vi "メイン.vi"() -> (2 "測定周期/ms":dbl, 3 "値転記用配列":T2[](array[typedef]))   [LabVIEW 2021] (continued)
                      n747 = property on="メイン測定ボタン_単発 8" class="Bool (指定)"("BoolText.Text"=w2025) -> ()  [unwired: 2 in, 2 out]
                      n748 = local write "csv入力項目min 8"(w2019) -> ()
                      n749 = local write "csv入力項目max 8"(w2020) -> ()
                      n750 = property on="メイン測定ボタン_連続 8" class="Bool (指定)"("Visible"=w2024) -> ()  [unwired: 2 in, 2 out]
                      n751 = property on="メイン測定ボタン_単発 8" class="Bool (指定)"("Visible"=w2023) -> ()  [unwired: 2 in, 2 out]
                    }
                    frame #2 {
                      # "⑯"
                      # "⑨"
                      # "⑧"
                      # "⑦"
                      # "⑥"
                      n752 = local read "メインON/OFF_\n設定 8"() -> (w2073:T1)
                      n753 = local write "メインON/OFF_\n保存確認 8"(w2073) -> ()
                      n754 = local read "メイン設定_設定 8"() -> (w2071:T2)
                      n755 = Unbundle By Name(w2071) -> ("測定画面表示ボタン"=w2070:bool)
                      n756 = case shown="FALSE" w2070 {
                        tunnel: [w2076 TRUE] -> w2072
                        frame False {
                          w2076 = FALSE
                          n757 = property on="メイン測定ボタン_単発 8" class="Bool (指定)"("Visible"=w2076) -> ()  [unwired: 2 in, 2 out]
                          n758 = property on="メイン測定ボタン_連続 8" class="Bool (指定)"("Visible"=w2076) -> ()  [unwired: 2 in, 2 out]
                        }
                        frame True {
                        }
                      }
                      n759 = local write "メインON/OFF_制御器 8"(w2073) -> ()
                      n760 = property on="メインON/OFF_制御器 8" class="Clust (指定)"("Visible"=w2072) -> ()  [unwired: 2 in, 2 out]
                      n761 = property on="メイン設定No_設定 8" class="Clust (指定)"("Visible"=w2072) -> ()  [unwired: 2 in, 2 out]
                      n762 = property on="メイン設定_設定 8" class="Clust (指定)"("Visible"=w2072) -> ()  [unwired: 2 in, 2 out]
                      n763 = property on="キャンセルボタン 8" class="Bool (指定)"("Visible"=w2072) -> ()  [unwired: 2 in, 2 out]
                    }
                  }
                  n764 = Replace Array Subset(array=w1852, new element=w1845, index=7) -> (w1851:T2[])
                }
                frame 8 {
                  # "⑱"
                  # "⑰"
                  # "2つ目の配列に転記"
                  # "32回繰り返す為、増やす場合はこのケースストラクチャーを複製する\n複製時、設定項目の配列やボタンも複製する為、下記のボタン類の移動はしない事"
                  # "iniからデータ読み取り"
                  n765 = flat-sequence {
                    tunnel: w2087 -> [w2113]
                    tunnel: w2086 -> [w2114]
                    tunnel: [w2091] -> w2083
                    tunnel: [w2090] -> w2082
                    tunnel: w2083 -> [w2260]
                    tunnel: w2082 -> [w2259]
                    tunnel: [w2260] -> w2081
                    tunnel: [w2259] -> w2080
                    tunnel: [w2307] -> w2088
                    tunnel: [w2308] -> w2089
                    tunnel: w2081 -> [w2308]
                    tunnel: w2080 -> [w2307]
                    tunnel: [w2304] -> w2078
                    frame #0 {
                      w2092 = "設定9"
                      # "複製時に変更する項目\n①②③④⑤⑥⑦⑧⑨　⑪⑫\nローカル変数\n⑬⑭\nセレクション\n⑮⑯\nプロパティノードが\n対象配列になっているか確認\n⑰\n指標値\n⑱\n複製したケースのTrue定数を削除"
                      # "⑭"
                      # "⑬"
                      # "⑫"
                      # "⑪"
                      # "④"
                      # "③"
                      # "setting.iniファイルからの設定項目の読み取り"
                      n766 = local read "メイン設定No_設定 9"() -> (w2110:T5)
                      n767 = call-poly <vilib>:"Read Key.vi"("section"="No9.", "error in (no error)"=w2114, "key"="No.", "refnum"=w2113) -> ("error out"=w2107:errorcluster, "value"=w2111:i32, "refnum out"=w2105:T10)  [unwired: 4 in, 1 out]
                      n768 = Bundle By Name(cluster=w2110, "No."=w2111) -> (w2112:T5)
                      n769 = local write "メイン設定No_設定 9"(w2112) -> ()
                      n770 = for {
                        shift-right: [w2122] -> w2109
                        shift-left: w2105 -> [w2123]
                        shift-right: [w2119] -> w2108
                        shift-left: w2107 -> [w2120]
                        tunnel: string[] ["規格", "規格上限", "規格下限", "ポートNo.", "測定モード", "規格単位", "品質チェック項目", "測定周期", "実測MAX", "実測MIN", "実測(MAX)", "実測(MIN)", "測定画面表示ボタン", "ゲージポートNo."] -> [w2118] mode=indexing
                        tunnel: w2092 -> [w2115]
                        i -> [w2121]
                        # "②"
                        # "①"
                        n771 = local read "メイン設定_設定 9"() -> (w2116:T2)
                        n772 = case shown="0, デフォルト" w2121 {
                          tunnel: w2123 -> [w2132 w2141 w2150 w2159 w2168 w2177 w2186 w2195 w2204 w2213 w2222 w2231 w2240 w2249]
                          tunnel: [w2131 w2140 w2149 w2158 w2167 w2176 w2185 w2194 w2203 w2212 w2221 w2230 w2239 w2248] -> w2122
                          tunnel: w2115 -> [w2130 w2139 w2148 w2157 w2166 w2175 w2184 w2193 w2202 w2211 w2220 w2229 w2238 w2247]
                          tunnel: w2120 -> [w2129 w2138 w2147 w2156 w2165 w2174 w2183 w2192 w2201 w2210 w2219 w2228 w2237 w2246]
                          tunnel: [w2128 w2137 w2146 w2155 w2164 w2173 w2182 w2191 w2200 w2209 w2218 w2227 w2236 w2245] -> w2119
                          tunnel: w2118 -> [_ _ _ _ _ w2171 _ _ _ _ _ _ _ _]
                          tunnel: w2118 -> [_ _ _ _ _ _ w2180 _ _ _ _ w2225 _ _]
                          tunnel: w2118 -> [w2126 w2135 w2144 w2153 w2162 _ _ w2189 w2198 w2207 w2216 _ w2234 w2243]
                          tunnel: [w2125 w2134 w2143 w2152 w2161 w2169 w2178 w2187 w2197 w2206 w2215 w2224 w2233 w2242] -> w2117
                          tunnel: w2116 -> [w2124 w2133 w2142 w2151 w2160 w2170 w2179 w2188 w2196 w2205 w2214 w2223 w2232 w2241]
                          frame 0, Default {
                            n773 = call-poly <vilib>:"Read Key.vi"("section"=w2130, "error in (no error)"=w2129, "key"=w2126, "refnum"=w2132) -> ("error out"=w2128:errorcluster, "value"=w2127:string, "refnum out"=w2131:T10)  [unwired: 4 in, 1 out]
                            n774 = Bundle By Name(cluster=w2124, "規格"=w2127) -> (w2125:T2)
                          }
                          frame 1 {
                            n775 = call-poly <vilib>:"Read Key.vi"("section"=w2139, "error in (no error)"=w2138, "key"=w2135, "refnum"=w2141) -> ("error out"=w2137:errorcluster, "value"=w2136:string, "refnum out"=w2140:T10)  [unwired: 4 in, 1 out]
                            n776 = Bundle By Name(cluster=w2133, "規格上限"=w2136) -> (w2134:T2)
                          }
                          frame 2 {
                            n777 = call-poly <vilib>:"Read Key.vi"("section"=w2148, "error in (no error)"=w2147, "key"=w2144, "refnum"=w2150) -> ("error out"=w2146:errorcluster, "value"=w2145:string, "refnum out"=w2149:T10)  [unwired: 4 in, 1 out]
                            n778 = Bundle By Name(cluster=w2142, "規格下限"=w2145) -> (w2143:T2)
                          }
                          frame 3 {
                            n779 = call-poly <vilib>:"Read Key.vi"("section"=w2157, "error in (no error)"=w2156, "key"=w2153, "refnum"=w2159) -> ("error out"=w2155:errorcluster, "value"=w2154:i32, "refnum out"=w2158:T10)  [unwired: 4 in, 1 out]
                            n780 = Bundle By Name(cluster=w2151, "ポートNo."=w2154) -> (w2152:T2)
                          }
                          frame 4 {
                            n781 = call-poly <vilib>:"Read Key.vi"("section"=w2166, "error in (no error)"=w2165, "key"=w2162, "refnum"=w2168) -> ("error out"=w2164:errorcluster, "value"=w2163:i32, "refnum out"=w2167:T10)  [unwired: 4 in, 1 out]
                            n782 = Bundle By Name(cluster=w2160, "測定モード"=w2163) -> (w2161:T2)
                          }
                          frame 5 {
                            n783 = call-poly <vilib>:"Read Key.vi"("section"=w2175, "error in (no error)"=w2174, "key"=w2171, "refnum"=w2177) -> ("error out"=w2173:errorcluster, "value"=w2172:string, "refnum out"=w2176:T10)  [unwired: 4 in, 1 out]
                            n784 = Bundle By Name(cluster=w2170, "規格単位"=w2172) -> (w2169:T2)
                          }
                          frame 6 {
                            n785 = call-poly <vilib>:"Read Key.vi"("section"=w2184, "error in (no error)"=w2183, "key"=w2180, "refnum"=w2186) -> ("error out"=w2182:errorcluster, "value"=w2181:string, "refnum out"=w2185:T10)  [unwired: 4 in, 1 out]
                            n786 = Bundle By Name(cluster=w2179, "品質チェック項目"=w2181) -> (w2178:T2)
                          }
                          frame 7 {
                            n787 = call-poly <vilib>:"Read Key.vi"("section"=w2193, "error in (no error)"=w2192, "key"=w2189, "refnum"=w2195) -> ("error out"=w2191:errorcluster, "value"=w2190:i32, "refnum out"=w2194:T10)  [unwired: 4 in, 1 out]
                            n788 = Bundle By Name(cluster=w2188, "測定周期"=w2190) -> (w2187:T2)
                          }
                          frame 8 {
                            n789 = call-poly <vilib>:"Read Key.vi"("section"=w2202, "error in (no error)"=w2201, "key"=w2198, "refnum"=w2204) -> ("error out"=w2200:errorcluster, "value"=w2199:string, "refnum out"=w2203:T10)  [unwired: 4 in, 1 out]
                            n790 = Bundle By Name(cluster=w2196, "実測値MAX"=w2199) -> (w2197:T2)
                          }
                          frame 9 {
                            n791 = call-poly <vilib>:"Read Key.vi"("section"=w2211, "error in (no error)"=w2210, "key"=w2207, "refnum"=w2213) -> ("error out"=w2209:errorcluster, "value"=w2208:string, "refnum out"=w2212:T10)  [unwired: 4 in, 1 out]
                            n792 = Bundle By Name(cluster=w2205, "実測値MIN"=w2208) -> (w2206:T2)
                          }
                          frame 10 {
                            n793 = call-poly <vilib>:"Read Key.vi"("section"=w2220, "error in (no error)"=w2219, "key"=w2216, "refnum"=w2222) -> ("error out"=w2218:errorcluster, "value"=w2217:string, "refnum out"=w2221:T10)  [unwired: 4 in, 1 out]
                            n794 = Bundle By Name(cluster=w2214, "実測値(MAX)"=w2217) -> (w2215:T2)
                          }
                          frame 11 {
                            n795 = call-poly <vilib>:"Read Key.vi"("section"=w2229, "error in (no error)"=w2228, "key"=w2225, "refnum"=w2231) -> ("error out"=w2227:errorcluster, "value"=w2226:string, "refnum out"=w2230:T10)  [unwired: 4 in, 1 out]
                            n796 = Bundle By Name(cluster=w2223, "実測値(MIN)"=w2226) -> (w2224:T2)
                          }
                          frame 12 {
                            n797 = call-poly <vilib>:"Read Key.vi"("section"=w2238, "error in (no error)"=w2237, "key"=w2234, "refnum"=w2240) -> ("error out"=w2236:errorcluster, "value"=w2235:bool, "refnum out"=w2239:T10)  [unwired: 4 in, 1 out]
                            n798 = Bundle By Name(cluster=w2232, "測定画面表示ボタン"=w2235) -> (w2233:T2)
                          }
                          frame 13 {
                            n799 = call-poly <vilib>:"Read Key.vi"("section"=w2247, "error in (no error)"=w2246, "key"=w2243, "refnum"=w2249) -> ("error out"=w2245:errorcluster, "value"=w2244:string, "refnum out"=w2248:T10)  [unwired: 4 in, 1 out]
                            n800 = Bundle By Name(cluster=w2241, "ゲージポートNo"=w2244) -> (w2242:T2)
                          }
                        }
                        n801 = local write "メイン設定_設定 9"(w2117) -> ()
                      }
                      n802 = local read "メインON/OFF_\n設定 9"() -> (w2101:T1)
                      n803 = call-poly <vilib>:"Read Key.vi"("section"=w2092, "error in (no error)"=w2108, "key"="使用ON/OFF", "refnum"=w2109) -> ("error out"=w2093:errorcluster, "value"=w2099:bool, "refnum out"=w2094:T10)  [unwired: 4 in, 1 out]
                      n804 = Bundle By Name(cluster=w2101, "使用ON/OFF"=w2099) -> (w2102:T1)
                      n805 = local write "メインON/OFF_\n設定 9"(w2102) -> ()
                      n806 = local read "CSV項目名 9"() -> (w2097:T3)
                      n807 = call-poly <vilib>:"Read Key.vi"("section"=w2092, "error in (no error)"=w2093, "key"="CSVヘッダー名", "refnum"=w2094) -> ("error out"=w2090:errorcluster, "value"=w2095:string, "refnum out"=w2091:T10)  [unwired: 4 in, 1 out]
                      n808 = Bundle By Name(cluster=w2097, "CSV項目名"=w2095) -> (w2096:T3)
                      n809 = local write "CSV項目名 9"(w2096) -> ()
                    }
                    frame #1 {
                      # "csvヘッダー項目作成"
                      # "⑮"
                      # "⑤"
                      n810 = local read "CSV項目名 9"() -> (w2254:T3)
                      n811 = Unbundle By Name(w2254) -> ("CSV項目名"=w2251:string)
                      n812 = local read "メイン設定_設定 9"() -> (w2255:T2)
                      n813 = Unbundle By Name(w2255) -> ("測定モード"=w2250:u16)
                      n814 = case shown="0, デフォルト" w2250 {
                        tunnel: ["単発測定" _ "多点測定"] -> w2258
                        tunnel: [FALSE TRUE FALSE] -> w2257
                        tunnel: [TRUE FALSE TRUE] -> w2256
                        frame 0, Default {
                        }
                        frame 1 {
                        }
                        frame 2 {
                        }
                      }
                      n815 = case shown="1" w2250 {
                        tunnel: w2251 -> [w2264 w2276 w2285]
                        tunnel: [w2262 w2274 w2287] -> w2253
                        tunnel: [w2261 w2273 w2286] -> w2252
                        frame 1 {
                          n816 = Empty String/Path?(string/path=w2264) -> (empty?=w2263:bool)
                          n817 = case shown="FALSE" w2263 {
                            tunnel: w2264 -> [w2270 _]
                            tunnel: w2264 -> [w2269 _]
                            tunnel: [w2266 ""] -> w2262
                            tunnel: [w2265 ""] -> w2261
                            frame False {
                              n818 = Concatenate Strings(w2270, "_max") -> (w2266:string)
                              n819 = Concatenate Strings(w2269, "_min") -> (w2265:string)
                            }
                            frame True {
                            }
                          }
                        }
                        frame 2 {
                          n820 = Empty String/Path?(string/path=w2276) -> (empty?=w2275:bool)
                          n821 = case shown="FALSE" w2275 {
                            tunnel: w2276 -> [w2282 _]
                            tunnel: w2276 -> [w2281 _]
                            tunnel: [w2278 ""] -> w2274
                            tunnel: [w2277 ""] -> w2273
                            frame False {
                              n822 = Concatenate Strings(w2282, "_max") -> (w2278:string)
                              n823 = Concatenate Strings(w2281, "_min") -> (w2277:string)
                            }
                            frame True {
                            }
                          }
                        }
                        frame 0, Default {
                          n824 = Empty String/Path?(string/path=w2285) -> (empty?=w2288:bool)
                          n825 = case shown="FALSE" w2288 {
                            tunnel: w2285 -> [w2292 _]
                            tunnel: [w2290 ""] -> w2287
                            tunnel: ["" ""] -> w2286
                            frame False {
                              n826 = Concatenate Strings(w2292, "_value") -> (w2290:string)
                            }
                            frame True {
                            }
                          }
                        }
                      }
                      n827 = property on="メイン測定ボタン_単発 9" class="Bool (指定)"("BoolText.Text"=w2258) -> ()  [unwired: 2 in, 2 out]
                      n828 = local write "csv入力項目min 9"(w2252) -> ()
                      n829 = local write "csv入力項目max 9"(w2253) -> ()
                      n830 = property on="メイン測定ボタン_連続 9" class="Bool (指定)"("Visible"=w2257) -> ()  [unwired: 2 in, 2 out]
                      n831 = property on="メイン測定ボタン_単発 9" class="Bool (指定)"("Visible"=w2256) -> ()  [unwired: 2 in, 2 out]
                    }
                    frame #2 {
                      # "⑯"
                      # "⑨"
                      # "⑧"
                      # "⑦"
                      # "⑥"
                      n832 = local read "メインON/OFF_\n設定 9"() -> (w2306:T1)
                      n833 = local write "メインON/OFF_\n保存確認 9"(w2306) -> ()
                      n834 = local read "メイン設定_設定 9"() -> (w2304:T2)
                      n835 = Unbundle By Name(w2304) -> ("測定画面表示ボタン"=w2303:bool)
                      n836 = case shown="FALSE" w2303 {
                        tunnel: [w2309 TRUE] -> w2305
                        frame False {
                          w2309 = FALSE
                          n837 = property on="メイン測定ボタン_単発 9" class="Bool (指定)"("Visible"=w2309) -> ()  [unwired: 2 in, 2 out]
                          n838 = property on="メイン測定ボタン_連続 9" class="Bool (指定)"("Visible"=w2309) -> ()  [unwired: 2 in, 2 out]
                        }
                        frame True {
                        }
                      }
                      n839 = local write "メインON/OFF_制御器 9"(w2306) -> ()
                      n840 = property on="メインON/OFF_制御器 9" class="Clust (指定)"("Visible"=w2305) -> ()  [unwired: 2 in, 2 out]
                      n841 = property on="メイン設定No_設定 9" class="Clust (指定)"("Visible"=w2305) -> ()  [unwired: 2 in, 2 out]
                      n842 = property on="メイン設定_設定 9" class="Clust (指定)"("Visible"=w2305) -> ()  [unwired: 2 in, 2 out]
                      n843 = property on="キャンセルボタン 9" class="Bool (指定)"("Visible"=w2305) -> ()  [unwired: 2 in, 2 out]
                    }
                  }
                  n844 = Replace Array Subset(array=w2085, new element=w2078, index=8) -> (w2084:T2[])
                }
                frame 9 {
                  # "⑱"
                  # "⑰"
                  # "2つ目の配列に転記"
                  # "32回繰り返す為、増やす場合はこのケースストラクチャーを複製する\n複製時、設定項目の配列やボタンも複製する為、下記のボタン類の移動はしない事"
                  # "iniからデータ読み取り"
                  n845 = flat-sequence {
                    tunnel: w2320 -> [w2346]
                    tunnel: w2319 -> [w2347]
                    tunnel: [w2325] -> w2316
                    tunnel: [w2324] -> w2315
                    tunnel: w2316 -> [w2493]
                    tunnel: w2315 -> [w2492]
                    tunnel: [w2493] -> w2314
                    tunnel: [w2492] -> w2313
                    tunnel: [w2540] -> w2321
                    tunnel: [w2541] -> w2322
                    tunnel: w2314 -> [w2541]
                    tunnel: w2313 -> [w2540]
                    tunnel: [w2537] -> w2311
                    frame #0 {
                      w2323 = "設定10"
                      # "複製時に変更する項目\n①②③④⑤⑥⑦⑧⑨　⑪⑫\nローカル変数\n⑬⑭\nセレクション\n⑮⑯\nプロパティノードが\n対象配列になっているか確認\n⑰\n指標値\n⑱\n複製したケースのTrue定数を削除"
                      # "⑭"
                      # "⑬"
                      # "⑫"
                      # "⑪"
                      # "④"
                      # "③"
                      # "setting.iniファイルからの設定項目の読み取り"
                      n846 = local read "メイン設定No_設定 10"() -> (w2343:T5)
                      n847 = call-poly <vilib>:"Read Key.vi"("section"="No10.", "error in (no error)"=w2347, "key"="No.", "refnum"=w2346) -> ("error out"=w2340:errorcluster, "value"=w2344:i32, "refnum out"=w2338:T10)  [unwired: 4 in, 1 out]
                      n848 = Bundle By Name(cluster=w2343, "No."=w2344) -> (w2345:T5)
                      n849 = local write "メイン設定No_設定 10"(w2345) -> ()
                      n850 = for {
                        shift-right: [w2355] -> w2342
                        shift-left: w2338 -> [w2356]
                        shift-right: [w2352] -> w2341
                        shift-left: w2340 -> [w2353]
                        tunnel: string[] ["規格", "規格上限", "規格下限", "ポートNo.", "測定モード", "規格単位", "品質チェック項目", "測定周期", "実測MAX", "実測MIN", "実測(MAX)", "実測(MIN)", "測定画面表示ボタン", "ゲージポートNo."] -> [w2351] mode=indexing
                        tunnel: w2323 -> [w2348]
                        i -> [w2354]
                        # "②"
                        # "①"
                        n851 = local read "メイン設定_設定 10"() -> (w2349:T2)
                        n852 = case shown="0, デフォルト" w2354 {
                          tunnel: w2356 -> [w2365 w2374 w2383 w2392 w2401 w2410 w2419 w2428 w2437 w2446 w2455 w2464 w2473 w2482]
                          tunnel: [w2364 w2373 w2382 w2391 w2400 w2409 w2418 w2427 w2436 w2445 w2454 w2463 w2472 w2481] -> w2355
                          tunnel: w2348 -> [w2363 w2372 w2381 w2390 w2399 w2408 w2417 w2426 w2435 w2444 w2453 w2462 w2471 w2480]
                          tunnel: w2353 -> [w2362 w2371 w2380 w2389 w2398 w2407 w2416 w2425 w2434 w2443 w2452 w2461 w2470 w2479]
                          tunnel: [w2361 w2370 w2379 w2388 w2397 w2406 w2415 w2424 w2433 w2442 w2451 w2460 w2469 w2478] -> w2352
                          tunnel: w2351 -> [_ _ _ _ _ w2404 _ _ _ _ _ _ _ _]
                          tunnel: w2351 -> [_ _ _ _ _ _ w2413 _ _ _ _ w2458 _ _]
                          tunnel: w2351 -> [w2359 w2368 w2377 w2386 w2395 _ _ w2422 w2431 w2440 w2449 _ w2467 w2476]
                          tunnel: [w2358 w2367 w2376 w2385 w2394 w2402 w2411 w2420 w2430 w2439 w2448 w2457 w2466 w2475] -> w2350
                          tunnel: w2349 -> [w2357 w2366 w2375 w2384 w2393 w2403 w2412 w2421 w2429 w2438 w2447 w2456 w2465 w2474]
                          frame 0, Default {
                            n853 = call-poly <vilib>:"Read Key.vi"("section"=w2363, "error in (no error)"=w2362, "key"=w2359, "refnum"=w2365) -> ("error out"=w2361:errorcluster, "value"=w2360:string, "refnum out"=w2364:T10)  [unwired: 4 in, 1 out]
                            n854 = Bundle By Name(cluster=w2357, "規格"=w2360) -> (w2358:T2)
                          }
                          frame 1 {
                            n855 = call-poly <vilib>:"Read Key.vi"("section"=w2372, "error in (no error)"=w2371, "key"=w2368, "refnum"=w2374) -> ("error out"=w2370:errorcluster, "value"=w2369:string, "refnum out"=w2373:T10)  [unwired: 4 in, 1 out]
                            n856 = Bundle By Name(cluster=w2366, "規格上限"=w2369) -> (w2367:T2)
                          }
                          frame 2 {
                            n857 = call-poly <vilib>:"Read Key.vi"("section"=w2381, "error in (no error)"=w2380, "key"=w2377, "refnum"=w2383) -> ("error out"=w2379:errorcluster, "value"=w2378:string, "refnum out"=w2382:T10)  [unwired: 4 in, 1 out]
                            n858 = Bundle By Name(cluster=w2375, "規格下限"=w2378) -> (w2376:T2)
                          }
                          frame 3 {
                            n859 = call-poly <vilib>:"Read Key.vi"("section"=w2390, "error in (no error)"=w2389, "key"=w2386, "refnum"=w2392) -> ("error out"=w2388:errorcluster, "value"=w2387:i32, "refnum out"=w2391:T10)  [unwired: 4 in, 1 out]
                            n860 = Bundle By Name(cluster=w2384, "ポートNo."=w2387) -> (w2385:T2)
                          }
                          frame 4 {
                            n861 = call-poly <vilib>:"Read Key.vi"("section"=w2399, "error in (no error)"=w2398, "key"=w2395, "refnum"=w2401) -> ("error out"=w2397:errorcluster, "value"=w2396:i32, "refnum out"=w2400:T10)  [unwired: 4 in, 1 out]
                            n862 = Bundle By Name(cluster=w2393, "測定モード"=w2396) -> (w2394:T2)
                          }
                          frame 5 {
                            n863 = call-poly <vilib>:"Read Key.vi"("section"=w2408, "error in (no error)"=w2407, "key"=w2404, "refnum"=w2410) -> ("error out"=w2406:errorcluster, "value"=w2405:string, "refnum out"=w2409:T10)  [unwired: 4 in, 1 out]
                            n864 = Bundle By Name(cluster=w2403, "規格単位"=w2405) -> (w2402:T2)
                          }
                          frame 6 {
                            n865 = call-poly <vilib>:"Read Key.vi"("section"=w2417, "error in (no error)"=w2416, "key"=w2413, "refnum"=w2419) -> ("error out"=w2415:errorcluster, "value"=w2414:string, "refnum out"=w2418:T10)  [unwired: 4 in, 1 out]
                            n866 = Bundle By Name(cluster=w2412, "品質チェック項目"=w2414) -> (w2411:T2)
                          }
                          frame 7 {
                            n867 = call-poly <vilib>:"Read Key.vi"("section"=w2426, "error in (no error)"=w2425, "key"=w2422, "refnum"=w2428) -> ("error out"=w2424:errorcluster, "value"=w2423:i32, "refnum out"=w2427:T10)  [unwired: 4 in, 1 out]
                            n868 = Bundle By Name(cluster=w2421, "測定周期"=w2423) -> (w2420:T2)
                          }
                          frame 8 {
                            n869 = call-poly <vilib>:"Read Key.vi"("section"=w2435, "error in (no error)"=w2434, "key"=w2431, "refnum"=w2437) -> ("error out"=w2433:errorcluster, "value"=w2432:string, "refnum out"=w2436:T10)  [unwired: 4 in, 1 out]
                            n870 = Bundle By Name(cluster=w2429, "実測値MAX"=w2432) -> (w2430:T2)
                          }
                          frame 9 {
                            n871 = call-poly <vilib>:"Read Key.vi"("section"=w2444, "error in (no error)"=w2443, "key"=w2440, "refnum"=w2446) -> ("error out"=w2442:errorcluster, "value"=w2441:string, "refnum out"=w2445:T10)  [unwired: 4 in, 1 out]
                            n872 = Bundle By Name(cluster=w2438, "実測値MIN"=w2441) -> (w2439:T2)
                          }
                          frame 10 {
                            n873 = call-poly <vilib>:"Read Key.vi"("section"=w2453, "error in (no error)"=w2452, "key"=w2449, "refnum"=w2455) -> ("error out"=w2451:errorcluster, "value"=w2450:string, "refnum out"=w2454:T10)  [unwired: 4 in, 1 out]
                            n874 = Bundle By Name(cluster=w2447, "実測値(MAX)"=w2450) -> (w2448:T2)
                          }
                          frame 11 {
                            n875 = call-poly <vilib>:"Read Key.vi"("section"=w2462, "error in (no error)"=w2461, "key"=w2458, "refnum"=w2464) -> ("error out"=w2460:errorcluster, "value"=w2459:string, "refnum out"=w2463:T10)  [unwired: 4 in, 1 out]
                            n876 = Bundle By Name(cluster=w2456, "実測値(MIN)"=w2459) -> (w2457:T2)
                          }
                          frame 12 {
                            n877 = call-poly <vilib>:"Read Key.vi"("section"=w2471, "error in (no error)"=w2470, "key"=w2467, "refnum"=w2473) -> ("error out"=w2469:errorcluster, "value"=w2468:bool, "refnum out"=w2472:T10)  [unwired: 4 in, 1 out]
                            n878 = Bundle By Name(cluster=w2465, "測定画面表示ボタン"=w2468) -> (w2466:T2)
                          }
                          frame 13 {
                            n879 = call-poly <vilib>:"Read Key.vi"("section"=w2480, "error in (no error)"=w2479, "key"=w2476, "refnum"=w2482) -> ("error out"=w2478:errorcluster, "value"=w2477:string, "refnum out"=w2481:T10)  [unwired: 4 in, 1 out]
                            n880 = Bundle By Name(cluster=w2474, "ゲージポートNo"=w2477) -> (w2475:T2)
                          }
                        }
                        n881 = local write "メイン設定_設定 10"(w2350) -> ()
                      }
                      n882 = local read "メインON/OFF_\n設定 10"() -> (w2334:T1)
                      n883 = call-poly <vilib>:"Read Key.vi"("section"=w2323, "error in (no error)"=w2341, "key"="使用ON/OFF", "refnum"=w2342) -> ("error out"=w2326:errorcluster, "value"=w2332:bool, "refnum out"=w2327:T10)  [unwired: 4 in, 1 out]
                      n884 = Bundle By Name(cluster=w2334, "使用ON/OFF"=w2332) -> (w2335:T1)
                      n885 = local write "メインON/OFF_\n設定 10"(w2335) -> ()
                      n886 = local read "CSV項目名 10"() -> (w2330:T3)
                      n887 = call-poly <vilib>:"Read Key.vi"("section"=w2323, "error in (no error)"=w2326, "key"="CSVヘッダー名", "refnum"=w2327) -> ("error out"=w2324:errorcluster, "value"=w2328:string, "refnum out"=w2325:T10)  [unwired: 4 in, 1 out]
                      n888 = Bundle By Name(cluster=w2330, "CSV項目名"=w2328) -> (w2329:T3)
                      n889 = local write "CSV項目名 10"(w2329) -> ()
                    }
                    frame #1 {
                      # "csvヘッダー項目作成"
                      # "⑮"
                      # "⑤"
                      n890 = local read "CSV項目名 10"() -> (w2487:T3)
                      n891 = Unbundle By Name(w2487) -> ("CSV項目名"=w2484:string)
                      n892 = local read "メイン設定_設定 10"() -> (w2488:T2)
                      n893 = Unbundle By Name(w2488) -> ("測定モード"=w2483:u16)
                      n894 = case shown="0, デフォルト" w2483 {
                        tunnel: ["単発測定" _ "多点測定"] -> w2491
                        tunnel: [FALSE TRUE FALSE] -> w2490
                        tunnel: [TRUE FALSE TRUE] -> w2489
                        frame 0, Default {
                        }
                        frame 1 {
                        }
                        frame 2 {
                        }
                      }
                      n895 = case shown="1" w2483 {
                        tunnel: w2484 -> [w2497 w2509 w2518]
                        tunnel: [w2495 w2507 w2520] -> w2486
                        tunnel: [w2494 w2506 w2519] -> w2485
                        frame 1 {
                          n896 = Empty String/Path?(string/path=w2497) -> (empty?=w2496:bool)
                          n897 = case shown="FALSE" w2496 {
                            tunnel: w2497 -> [w2503 _]
                            tunnel: w2497 -> [w2502 _]
                            tunnel: [w2499 ""] -> w2495
                            tunnel: [w2498 ""] -> w2494
                            frame False {
                              n898 = Concatenate Strings(w2503, "_max") -> (w2499:string)
                              n899 = Concatenate Strings(w2502, "_min") -> (w2498:string)
                            }
                            frame True {
                            }
                          }
                        }
                        frame 2 {
                          n900 = Empty String/Path?(string/path=w2509) -> (empty?=w2508:bool)
                          n901 = case shown="FALSE" w2508 {
                            tunnel: w2509 -> [w2515 _]
                            tunnel: w2509 -> [w2514 _]
                            tunnel: [w2511 ""] -> w2507
                            tunnel: [w2510 ""] -> w2506
                            frame False {
                              n902 = Concatenate Strings(w2515, "_max") -> (w2511:string)
                              n903 = Concatenate Strings(w2514, "_min") -> (w2510:string)
                            }
                            frame True {
                            }
                          }
                        }
                        frame 0, Default {
                          n904 = Empty String/Path?(string/path=w2518) -> (empty?=w2521:bool)
                          n905 = case shown="FALSE" w2521 {
                            tunnel: w2518 -> [w2525 _]
                            tunnel: [w2523 ""] -> w2520
                            tunnel: ["" ""] -> w2519
                            frame False {
                              n906 = Concatenate Strings(w2525, "_value") -> (w2523:string)
                            }
                            frame True {
                            }
                          }
                        }
                      }
                      n907 = property on="メイン測定ボタン_単発 10" class="Bool (指定)"("BoolText.Text"=w2491) -> ()  [unwired: 2 in, 2 out]
                      n908 = local write "csv入力項目min 10"(w2485) -> ()
                      n909 = local write "csv入力項目max 10"(w2486) -> ()
                      n910 = property on="メイン測定ボタン_連続 10" class="Bool (指定)"("Visible"=w2490) -> ()  [unwired: 2 in, 2 out]
                      n911 = property on="メイン測定ボタン_単発 10" class="Bool (指定)"("Visible"=w2489) -> ()  [unwired: 2 in, 2 out]
                    }
                    frame #2 {
                      # "⑯"
                      # "⑨"
                      # "⑧"
                      # "⑦"
                      # "⑥"
                      n912 = local read "メインON/OFF_\n設定 10"() -> (w2539:T1)
                      n913 = local write "メインON/OFF_\n保存確認 10"(w2539) -> ()
                      n914 = local read "メイン設定_設定 10"() -> (w2537:T2)
                      n915 = Unbundle By Name(w2537) -> ("測定画面表示ボタン"=w2536:bool)
                      n916 = case shown="FALSE" w2536 {
                        tunnel: [w2542 TRUE] -> w2538
                        frame False {
                          w2542 = FALSE
                          n917 = property on="メイン測定ボタン_単発 10" class="Bool (指定)"("Visible"=w2542) -> ()  [unwired: 2 in, 2 out]
                          n918 = property on="メイン測定ボタン_連続 10" class="Bool (指定)"("Visible"=w2542) -> ()  [unwired: 2 in, 2 out]
                        }
                        frame True {
                        }
                      }
                      n919 = local write "メインON/OFF_制御器 10"(w2539) -> ()
                      n920 = property on="メインON/OFF_制御器 10" class="Clust (指定)"("Visible"=w2538) -> ()  [unwired: 2 in, 2 out]
                      n921 = property on="メイン設定No_設定 10" class="Clust (指定)"("Visible"=w2538) -> ()  [unwired: 2 in, 2 out]
                      n922 = property on="メイン設定_設定 10" class="Clust (指定)"("Visible"=w2538) -> ()  [unwired: 2 in, 2 out]
                      n923 = property on="キャンセルボタン 10" class="Bool (指定)"("Visible"=w2538) -> ()  [unwired: 2 in, 2 out]
                    }
                  }
                  n924 = Replace Array Subset(array=w2318, new element=w2311, index=9) -> (w2317:T2[])
                }
                frame 10 {
                  # "⑱"
                  # "⑰"
                  # "2つ目の配列に転記"
                  # "32回繰り返す為、増やす場合はこのケースストラクチャーを複製する\n複製時、設定項目の配列やボタンも複製する為、下記のボタン類の移動はしない事"
                  # "iniからデータ読み取り"
                  n925 = flat-sequence {
                    tunnel: w2553 -> [w2579]
                    tunnel: w2552 -> [w2580]
                    tunnel: [w2557] -> w2549
                    tunnel: [w2556] -> w2548
                    tunnel: w2549 -> [w2726]
                    tunnel: w2548 -> [w2725]
                    tunnel: [w2726] -> w2547
                    tunnel: [w2725] -> w2546
                    tunnel: [w2773] -> w2554
                    tunnel: [w2774] -> w2555
                    tunnel: w2547 -> [w2774]
                    tunnel: w2546 -> [w2773]
                    tunnel: [w2770] -> w2544
                    frame #0 {
                      w2558 = "設定11"
                      # "複製時に変更する項目\n①②③④⑤⑥⑦⑧⑨　⑪⑫\nローカル変数\n⑬⑭\nセレクション\n⑮⑯\nプロパティノードが\n対象配列になっているか確認\n⑰\n指標値\n⑱\n複製したケースのTrue定数を削除"
                      # "⑭"
                      # "⑬"
                      # "⑫"
                      # "⑪"
                      # "④"
                      # "③"
                      # "setting.iniファイルからの設定項目の読み取り"
                      n926 = local read "メイン設定No_設定 11"() -> (w2576:T5)
                      n927 = call-poly <vilib>:"Read Key.vi"("section"="No11.", "error in (no error)"=w2580, "key"="No.", "refnum"=w2579) -> ("error out"=w2573:errorcluster, "value"=w2577:i32, "refnum out"=w2571:T10)  [unwired: 4 in, 1 out]
                      n928 = Bundle By Name(cluster=w2576, "No."=w2577) -> (w2578:T5)
                      n929 = local write "メイン設定No_設定 11"(w2578) -> ()
                      n930 = for {
                        shift-right: [w2588] -> w2575
                        shift-left: w2571 -> [w2589]
                        shift-right: [w2585] -> w2574
                        shift-left: w2573 -> [w2586]
                        tunnel: string[] ["規格", "規格上限", "規格下限", "ポートNo.", "測定モード", "規格単位", "品質チェック項目", "測定周期", "実測MAX", "実測MIN", "実測(MAX)", "実測(MIN)", "測定画面表示ボタン", "ゲージポートNo."] -> [w2584] mode=indexing
                        tunnel: w2558 -> [w2581]
                        i -> [w2587]
                        # "②"
                        # "①"
                        n931 = local read "メイン設定_設定 11"() -> (w2582:T2)
                        n932 = case shown="0, デフォルト" w2587 {
                          tunnel: w2589 -> [w2598 w2607 w2616 w2625 w2634 w2643 w2652 w2661 w2670 w2679 w2688 w2697 w2706 w2715]
                          tunnel: [w2597 w2606 w2615 w2624 w2633 w2642 w2651 w2660 w2669 w2678 w2687 w2696 w2705 w2714] -> w2588
                          tunnel: w2581 -> [w2596 w2605 w2614 w2623 w2632 w2641 w2650 w2659 w2668 w2677 w2686 w2695 w2704 w2713]
                          tunnel: w2586 -> [w2595 w2604 w2613 w2622 w2631 w2640 w2649 w2658 w2667 w2676 w2685 w2694 w2703 w2712]
                          tunnel: [w2594 w2603 w2612 w2621 w2630 w2639 w2648 w2657 w2666 w2675 w2684 w2693 w2702 w2711] -> w2585
                          tunnel: w2584 -> [_ _ _ _ _ w2637 _ _ _ _ _ _ _ _]
                          tunnel: w2584 -> [_ _ _ _ _ _ w2646 _ _ _ _ w2691 _ _]
                          tunnel: w2584 -> [w2592 w2601 w2610 w2619 w2628 _ _ w2655 w2664 w2673 w2682 _ w2700 w2709]
                          tunnel: [w2591 w2600 w2609 w2618 w2627 w2635 w2644 w2653 w2663 w2672 w2681 w2690 w2699 w2708] -> w2583
                          tunnel: w2582 -> [w2590 w2599 w2608 w2617 w2626 w2636 w2645 w2654 w2662 w2671 w2680 w2689 w2698 w2707]
                          frame 0, Default {
                            n933 = call-poly <vilib>:"Read Key.vi"("section"=w2596, "error in (no error)"=w2595, "key"=w2592, "refnum"=w2598) -> ("error out"=w2594:errorcluster, "value"=w2593:string, "refnum out"=w2597:T10)  [unwired: 4 in, 1 out]
                            n934 = Bundle By Name(cluster=w2590, "規格"=w2593) -> (w2591:T2)
                          }
                          frame 1 {
                            n935 = call-poly <vilib>:"Read Key.vi"("section"=w2605, "error in (no error)"=w2604, "key"=w2601, "refnum"=w2607) -> ("error out"=w2603:errorcluster, "value"=w2602:string, "refnum out"=w2606:T10)  [unwired: 4 in, 1 out]
                            n936 = Bundle By Name(cluster=w2599, "規格上限"=w2602) -> (w2600:T2)
                          }
                          frame 2 {
                            n937 = call-poly <vilib>:"Read Key.vi"("section"=w2614, "error in (no error)"=w2613, "key"=w2610, "refnum"=w2616) -> ("error out"=w2612:errorcluster, "value"=w2611:string, "refnum out"=w2615:T10)  [unwired: 4 in, 1 out]
                            n938 = Bundle By Name(cluster=w2608, "規格下限"=w2611) -> (w2609:T2)
                          }
                          frame 3 {
                            n939 = call-poly <vilib>:"Read Key.vi"("section"=w2623, "error in (no error)"=w2622, "key"=w2619, "refnum"=w2625) -> ("error out"=w2621:errorcluster, "value"=w2620:i32, "refnum out"=w2624:T10)  [unwired: 4 in, 1 out]
                            n940 = Bundle By Name(cluster=w2617, "ポートNo."=w2620) -> (w2618:T2)
                          }
                          frame 4 {
                            n941 = call-poly <vilib>:"Read Key.vi"("section"=w2632, "error in (no error)"=w2631, "key"=w2628, "refnum"=w2634) -> ("error out"=w2630:errorcluster, "value"=w2629:i32, "refnum out"=w2633:T10)  [unwired: 4 in, 1 out]
                            n942 = Bundle By Name(cluster=w2626, "測定モード"=w2629) -> (w2627:T2)
                          }
                          frame 5 {
                            n943 = call-poly <vilib>:"Read Key.vi"("section"=w2641, "error in (no error)"=w2640, "key"=w2637, "refnum"=w2643) -> ("error out"=w2639:errorcluster, "value"=w2638:string, "refnum out"=w2642:T10)  [unwired: 4 in, 1 out]
                            n944 = Bundle By Name(cluster=w2636, "規格単位"=w2638) -> (w2635:T2)
                          }
                          frame 6 {
                            n945 = call-poly <vilib>:"Read Key.vi"("section"=w2650, "error in (no error)"=w2649, "key"=w2646, "refnum"=w2652) -> ("error out"=w2648:errorcluster, "value"=w2647:string, "refnum out"=w2651:T10)  [unwired: 4 in, 1 out]
                            n946 = Bundle By Name(cluster=w2645, "品質チェック項目"=w2647) -> (w2644:T2)
                          }
                          frame 7 {
                            n947 = call-poly <vilib>:"Read Key.vi"("section"=w2659, "error in (no error)"=w2658, "key"=w2655, "refnum"=w2661) -> ("error out"=w2657:errorcluster, "value"=w2656:i32, "refnum out"=w2660:T10)  [unwired: 4 in, 1 out]
                            n948 = Bundle By Name(cluster=w2654, "測定周期"=w2656) -> (w2653:T2)
                          }
                          frame 8 {
                            n949 = call-poly <vilib>:"Read Key.vi"("section"=w2668, "error in (no error)"=w2667, "key"=w2664, "refnum"=w2670) -> ("error out"=w2666:errorcluster, "value"=w2665:string, "refnum out"=w2669:T10)  [unwired: 4 in, 1 out]
                            n950 = Bundle By Name(cluster=w2662, "実測値MAX"=w2665) -> (w2663:T2)
                          }
                          frame 9 {
                            n951 = call-poly <vilib>:"Read Key.vi"("section"=w2677, "error in (no error)"=w2676, "key"=w2673, "refnum"=w2679) -> ("error out"=w2675:errorcluster, "value"=w2674:string, "refnum out"=w2678:T10)  [unwired: 4 in, 1 out]
                            n952 = Bundle By Name(cluster=w2671, "実測値MIN"=w2674) -> (w2672:T2)
                          }
                          frame 10 {
                            n953 = call-poly <vilib>:"Read Key.vi"("section"=w2686, "error in (no error)"=w2685, "key"=w2682, "refnum"=w2688) -> ("error out"=w2684:errorcluster, "value"=w2683:string, "refnum out"=w2687:T10)  [unwired: 4 in, 1 out]
                            n954 = Bundle By Name(cluster=w2680, "実測値(MAX)"=w2683) -> (w2681:T2)
                          }
                          frame 11 {
                            n955 = call-poly <vilib>:"Read Key.vi"("section"=w2695, "error in (no error)"=w2694, "key"=w2691, "refnum"=w2697) -> ("error out"=w2693:errorcluster, "value"=w2692:string, "refnum out"=w2696:T10)  [unwired: 4 in, 1 out]
                            n956 = Bundle By Name(cluster=w2689, "実測値(MIN)"=w2692) -> (w2690:T2)
                          }
                          frame 12 {
                            n957 = call-poly <vilib>:"Read Key.vi"("section"=w2704, "error in (no error)"=w2703, "key"=w2700, "refnum"=w2706) -> ("error out"=w2702:errorcluster, "value"=w2701:bool, "refnum out"=w2705:T10)  [unwired: 4 in, 1 out]
                            n958 = Bundle By Name(cluster=w2698, "測定画面表示ボタン"=w2701) -> (w2699:T2)
                          }
                          frame 13 {
                            n959 = call-poly <vilib>:"Read Key.vi"("section"=w2713, "error in (no error)"=w2712, "key"=w2709, "refnum"=w2715) -> ("error out"=w2711:errorcluster, "value"=w2710:string, "refnum out"=w2714:T10)  [unwired: 4 in, 1 out]
                            n960 = Bundle By Name(cluster=w2707, "ゲージポートNo"=w2710) -> (w2708:T2)
                          }
                        }
                        n961 = local write "メイン設定_設定 11"(w2583) -> ()
                      }
                      n962 = local read "メインON/OFF_\n設定 11"() -> (w2567:T1)
                      n963 = call-poly <vilib>:"Read Key.vi"("section"=w2558, "error in (no error)"=w2574, "key"="使用ON/OFF", "refnum"=w2575) -> ("error out"=w2559:errorcluster, "value"=w2565:bool, "refnum out"=w2560:T10)  [unwired: 4 in, 1 out]
                      n964 = Bundle By Name(cluster=w2567, "使用ON/OFF"=w2565) -> (w2568:T1)
                      n965 = local write "メインON/OFF_\n設定 11"(w2568) -> ()
                      n966 = local read "CSV項目名 11"() -> (w2563:T3)
                      n967 = call-poly <vilib>:"Read Key.vi"("section"=w2558, "error in (no error)"=w2559, "key"="CSVヘッダー名", "refnum"=w2560) -> ("error out"=w2556:errorcluster, "value"=w2561:string, "refnum out"=w2557:T10)  [unwired: 4 in, 1 out]
                      n968 = Bundle By Name(cluster=w2563, "CSV項目名"=w2561) -> (w2562:T3)
                      n969 = local write "CSV項目名 11"(w2562) -> ()
                    }
                    frame #1 {
                      # "csvヘッダー項目作成"
                      # "⑮"
                      # "⑤"
                      n970 = local read "CSV項目名 11"() -> (w2720:T3)
                      n971 = Unbundle By Name(w2720) -> ("CSV項目名"=w2717:string)
                      n972 = local read "メイン設定_設定 11"() -> (w2721:T2)
                      n973 = Unbundle By Name(w2721) -> ("測定モード"=w2716:u16)
                      n974 = case shown="0, デフォルト" w2716 {
                        tunnel: ["単発測定" _ "多点測定"] -> w2724
                        tunnel: [FALSE TRUE FALSE] -> w2723
                        tunnel: [TRUE FALSE TRUE] -> w2722
                        frame 0, Default {
                        }
                        frame 1 {
                        }
                        frame 2 {
                        }
                      }
                      n975 = case shown="1" w2716 {
                        tunnel: w2717 -> [w2730 w2742 w2751]
                        tunnel: [w2728 w2740 w2753] -> w2719
                        tunnel: [w2727 w2739 w2752] -> w2718
                        frame 1 {
                          n976 = Empty String/Path?(string/path=w2730) -> (empty?=w2729:bool)
                          n977 = case shown="FALSE" w2729 {
                            tunnel: w2730 -> [w2736 _]
                            tunnel: w2730 -> [w2735 _]
                            tunnel: [w2732 ""] -> w2728
                            tunnel: [w2731 ""] -> w2727
                            frame False {
                              n978 = Concatenate Strings(w2736, "_max") -> (w2732:string)
                              n979 = Concatenate Strings(w2735, "_min") -> (w2731:string)
                            }
                            frame True {
                            }
                          }
                        }
                        frame 2 {
                          n980 = Empty String/Path?(string/path=w2742) -> (empty?=w2741:bool)
                          n981 = case shown="FALSE" w2741 {
                            tunnel: w2742 -> [w2748 _]
                            tunnel: w2742 -> [w2747 _]
                            tunnel: [w2744 ""] -> w2740
                            tunnel: [w2743 ""] -> w2739
                            frame False {
                              n982 = Concatenate Strings(w2748, "_max") -> (w2744:string)
                              n983 = Concatenate Strings(w2747, "_min") -> (w2743:string)
                            }
                            frame True {
                            }
                          }
                        }
                        frame 0, Default {
                          n984 = Empty String/Path?(string/path=w2751) -> (empty?=w2754:bool)
                          n985 = case shown="FALSE" w2754 {
                            tunnel: w2751 -> [w2758 _]
                            tunnel: [w2756 ""] -> w2753
                            tunnel: ["" ""] -> w2752
                            frame False {
                              n986 = Concatenate Strings(w2758, "_value") -> (w2756:string)
                            }
                            frame True {
                            }
                          }
                        }
                      }
                      n987 = property on="メイン測定ボタン_単発 11" class="Bool (指定)"("BoolText.Text"=w2724) -> ()  [unwired: 2 in, 2 out]
                      n988 = local write "csv入力項目min 11"(w2718) -> ()
                      n989 = local write "csv入力項目max 11"(w2719) -> ()
                      n990 = property on="メイン測定ボタン_連続 11" class="Bool (指定)"("Visible"=w2723) -> ()  [unwired: 2 in, 2 out]
                      n991 = property on="メイン測定ボタン_単発 11" class="Bool (指定)"("Visible"=w2722) -> ()  [unwired: 2 in, 2 out]
                    }
                    frame #2 {
                      # "⑯"
                      # "⑨"
                      # "⑧"
                      # "⑦"
                      # "⑥"
                      n992 = local read "メインON/OFF_\n設定 11"() -> (w2772:T1)
                      n993 = local write "メインON/OFF_\n保存確認 11"(w2772) -> ()
                      n994 = local read "メイン設定_設定 11"() -> (w2770:T2)
                      n995 = Unbundle By Name(w2770) -> ("測定画面表示ボタン"=w2769:bool)
                      n996 = case shown="FALSE" w2769 {
                        tunnel: [w2775 TRUE] -> w2771
                        frame False {
                          w2775 = FALSE
                          n997 = property on="メイン測定ボタン_単発 11" class="Bool (指定)"("Visible"=w2775) -> ()  [unwired: 2 in, 2 out]
                          n998 = property on="メイン測定ボタン_連続 11" class="Bool (指定)"("Visible"=w2775) -> ()  [unwired: 2 in, 2 out]
                        }
                        frame True {
                        }
                      }
                      n999 = local write "メインON/OFF_制御器 11"(w2772) -> ()
                      n1000 = property on="メインON/OFF_制御器 11" class="Clust (指定)"("Visible"=w2771) -> ()  [unwired: 2 in, 2 out]
                      n1001 = property on="メイン設定No_設定 11" class="Clust (指定)"("Visible"=w2771) -> ()  [unwired: 2 in, 2 out]
                      n1002 = property on="メイン設定_設定 11" class="Clust (指定)"("Visible"=w2771) -> ()  [unwired: 2 in, 2 out]
                      n1003 = property on="キャンセルボタン 11" class="Bool (指定)"("Visible"=w2771) -> ()  [unwired: 2 in, 2 out]
                    }
                  }
                  n1004 = Replace Array Subset(array=w2551, new element=w2544, index=10) -> (w2550:T2[])
                }
                frame 11 {
                  # "⑱"
                  # "⑰"
                  # "2つ目の配列に転記"
                  # "32回繰り返す為、増やす場合はこのケースストラクチャーを複製する\n複製時、設定項目の配列やボタンも複製する為、下記のボタン類の移動はしない事"
                  # "iniからデータ読み取り"
                  n1005 = flat-sequence {
                    tunnel: w2787 -> [w2813]
                    tunnel: w2786 -> [w2814]
                    tunnel: [w2792] -> w2782
                    tunnel: [w2791] -> w2781
                    tunnel: w2782 -> [w2960]
                    tunnel: w2781 -> [w2959]
                    tunnel: [w2960] -> w2780
                    tunnel: [w2959] -> w2779
                    tunnel: [w3007] -> w2788
                    tunnel: [w3008] -> w2789
                    tunnel: w2780 -> [w3008]
                    tunnel: w2779 -> [w3007]
                    tunnel: [w3004] -> w2777
                    frame #0 {
                      w2790 = "設定12"
                      # "複製時に変更する項目\n①②③④⑤⑥⑦⑧⑨　⑪⑫\nローカル変数\n⑬⑭\nセレクション\n⑮⑯\nプロパティノードが\n対象配列になっているか確認\n⑰\n指標値\n⑱\n複製したケースのTrue定数を削除"
                      # "⑭"
                      # "⑬"
                      # "⑫"
                      # "⑪"
                      # "④"
                      # "③"
                      # "setting.iniファイルからの設定項目の読み取り"
                      n1006 = local read "メイン設定No_設定 12"() -> (w2810:T5)
                      n1007 = call-poly <vilib>:"Read Key.vi"("section"="No12.", "error in (no error)"=w2814, "key"="No.", "refnum"=w2813) -> ("error out"=w2807:errorcluster, "value"=w2811:i32, "refnum out"=w2805:T10)  [unwired: 4 in, 1 out]
                      n1008 = Bundle By Name(cluster=w2810, "No."=w2811) -> (w2812:T5)
                      n1009 = local write "メイン設定No_設定 12"(w2812) -> ()
                      n1010 = for {
                        shift-right: [w2822] -> w2809
                        shift-left: w2805 -> [w2823]
                        shift-right: [w2819] -> w2808
                        shift-left: w2807 -> [w2820]
                        tunnel: string[] ["規格", "規格上限", "規格下限", "ポートNo.", "測定モード", "規格単位", "品質チェック項目", "測定周期", "実測MAX", "実測MIN", "実測(MAX)", "実測(MIN)", "測定画面表示ボタン", "ゲージポートNo."] -> [w2818] mode=indexing
                        tunnel: w2790 -> [w2815]
                        i -> [w2821]
                        # "②"
                        # "①"
                        n1011 = local read "メイン設定_設定 12"() -> (w2816:T2)
                        n1012 = case shown="0, デフォルト" w2821 {
                          tunnel: w2823 -> [w2832 w2841 w2850 w2859 w2868 w2877 w2886 w2895 w2904 w2913 w2922 w2931 w2940 w2949]
                          tunnel: [w2831 w2840 w2849 w2858 w2867 w2876 w2885 w2894 w2903 w2912 w2921 w2930 w2939 w2948] -> w2822
                          tunnel: w2815 -> [w2830 w2839 w2848 w2857 w2866 w2875 w2884 w2893 w2902 w2911 w2920 w2929 w2938 w2947]
                          tunnel: w2820 -> [w2829 w2838 w2847 w2856 w2865 w2874 w2883 w2892 w2901 w2910 w2919 w2928 w2937 w2946]
                          tunnel: [w2828 w2837 w2846 w2855 w2864 w2873 w2882 w2891 w2900 w2909 w2918 w2927 w2936 w2945] -> w2819
                          tunnel: w2818 -> [_ _ _ _ _ w2871 _ _ _ _ _ _ _ _]
                          tunnel: w2818 -> [_ _ _ _ _ _ w2880 _ _ _ _ w2925 _ _]
                          tunnel: w2818 -> [w2826 w2835 w2844 w2853 w2862 _ _ w2889 w2898 w2907 w2916 _ w2934 w2943]
                          tunnel: [w2825 w2834 w2843 w2852 w2861 w2869 w2878 w2887 w2897 w2906 w2915 w2924 w2933 w2942] -> w2817
                          tunnel: w2816 -> [w2824 w2833 w2842 w2851 w2860 w2870 w2879 w2888 w2896 w2905 w2914 w2923 w2932 w2941]
                          frame 0, Default {
                            n1013 = call-poly <vilib>:"Read Key.vi"("section"=w2830, "error in (no error)"=w2829, "key"=w2826, "refnum"=w2832) -> ("error out"=w2828:errorcluster, "value"=w2827:string, "refnum out"=w2831:T10)  [unwired: 4 in, 1 out]
                            n1014 = Bundle By Name(cluster=w2824, "規格"=w2827) -> (w2825:T2)
                          }
                          frame 1 {
                            n1015 = call-poly <vilib>:"Read Key.vi"("section"=w2839, "error in (no error)"=w2838, "key"=w2835, "refnum"=w2841) -> ("error out"=w2837:errorcluster, "value"=w2836:string, "refnum out"=w2840:T10)  [unwired: 4 in, 1 out]
                            n1016 = Bundle By Name(cluster=w2833, "規格上限"=w2836) -> (w2834:T2)
                          }
                          frame 2 {
                            n1017 = call-poly <vilib>:"Read Key.vi"("section"=w2848, "error in (no error)"=w2847, "key"=w2844, "refnum"=w2850) -> ("error out"=w2846:errorcluster, "value"=w2845:string, "refnum out"=w2849:T10)  [unwired: 4 in, 1 out]
                            n1018 = Bundle By Name(cluster=w2842, "規格下限"=w2845) -> (w2843:T2)
                          }
                          frame 3 {
